vi "User data_Cnsl.vi"(6 "Error In":errorcluster, 9 "refnum in":refnum<file>) -> (0 "error out":errorcluster, 3 "refnum out":refnum<file>)   [LabVIEW 2018]
uses:
  Global_1259.vi
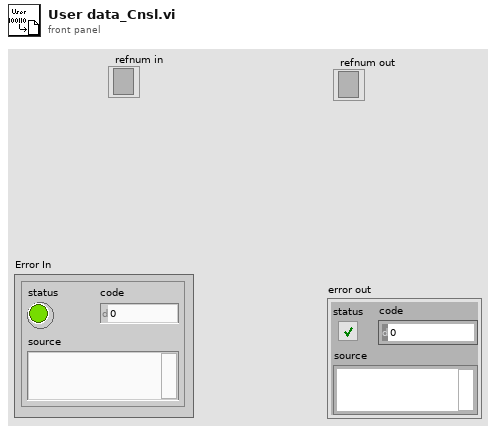
[diagram p1: front panel]
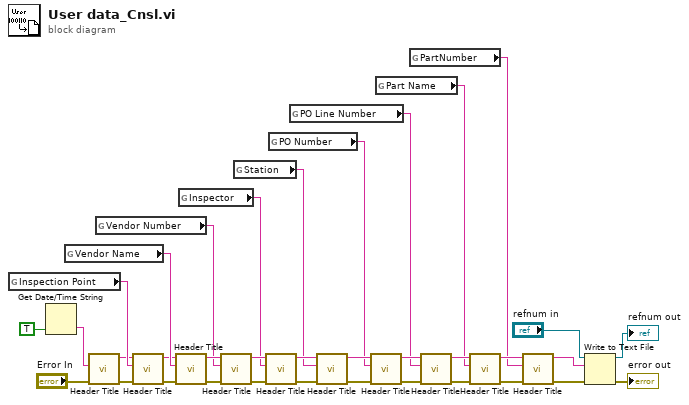
[diagram p0: block diagram]
diagram:
  n1 = global read "Global_1259.vi" "Inspection Point"() -> (w5:string)
  n2 = Get Date/Time String(want seconds? (F)=TRUE) -> (time string=w23:string)  [unwired: 2 in, 1 out]
  n3 = global read "Global_1259.vi" "Vendor Name"() -> (w13:string)
  n4 = call "Header Title.vi"("Error In"="Error In", "Header Title"=w23) -> ("Error Out"=w2:errorcluster, "String out"=w4:string)  [unwired: 8 in]
  n5 = global read "Global_1259.vi" "Vendor Number"() -> (w12:string)
  n6 = call "Header Title.vi"("Error In"=w2, "Header Title"=w5, "String in"=w4) -> ("Error Out"=w1:errorcluster, "String out"=w3:string)  [unwired: 7 in]
  n7 = call "Header Title.vi"("Error In"=w1, "Header Title"=w13, "String in"=w3) -> ("Error Out"=w29:errorcluster, "String out"=w33:string)  [unwired: 7 in]
  n8 = global read "Global_1259.vi" "Inspector"() -> (w11:string)
  n9 = call "Header Title.vi"("Error In"=w29, "Header Title"=w12, "String in"=w33) -> ("Error Out"=w28:errorcluster, "String out"=w30:string)  [unwired: 7 in]
  n10 = global read "Global_1259.vi" "Station"() -> (w10:string)
  n11 = call "Header Title.vi"("Error In"=w28, "Header Title"=w11, "String in"=w30) -> ("Error Out"=w27:errorcluster, "String out"=w32:string)  [unwired: 7 in]
  n12 = global read "Global_1259.vi" "PO Number"() -> (w9:string)
  n13 = global read "Global_1259.vi" "PO Line Number"() -> (w8:string)
  n14 = call "Header Title.vi"("Error In"=w27, "Header Title"=w10, "String in"=w32) -> ("Error Out"=w26:errorcluster, "String out"=w31:string)  [unwired: 7 in]
  n15 = call "Header Title.vi"("Error In"=w26, "Header Title"=w9, "String in"=w31) -> ("Error Out"=w16:errorcluster, "String out"=w17:string)  [unwired: 7 in]
  n16 = global read "Global_1259.vi" "Part Name"() -> (w7:string)
  n17 = global read "Global_1259.vi" "PartNumber"() -> (w6:string)
  n18 = call "Header Title.vi"("Error In"=w16, "Header Title"=w8, "String in"=w17) -> ("Error Out"=w14:errorcluster, "String out"=w15:string)  [unwired: 7 in]
  n19 = call "Header Title.vi"("Error In"=w14, "Header Title"=w7, "String in"=w15) -> ("Error Out"=w24:errorcluster, "String out"=w25:string)  [unwired: 7 in]
  n20 = call "Header Title.vi"("Error In"=w24, "Header Title"=w6, "String in"=w25) -> ("Error Out"=w19:errorcluster, "String out"=w20:string)  [unwired: 7 in]
  n21 = Write to Text File(file (use dialog)="refnum in", text=w20, error in=w19) -> (refnum out=→"refnum out":refnum<file>, error out=→"error out":errorcluster)  [unwired: 1 in, 1 out]
